vi "Delete Logged Files.vi"() -> ()   [LabVIEW 2019]
uses:
  <vilib>/Skyline/File/File/NI Skyline File.lvclass
  C:/Program Files (x86)/National Instruments/LabVIEW 2019/vi.lib/Skyline/File/Base/NI Skyline File Base.lvclass
  <vilib>/Skyline/File/Filter/Create Filter (Name).vi
  <vilib>/Skyline/File/Filter/Create Filter (Extension).vi
  <vilib>/Skyline/File/File/Query Files.vi
  <vilib>/Skyline/File/File/Delete (Multiple).vi
  <vilib>/Skyline/File/Filter/NI Skyline File Filter.lvclass
  <vilib>/Skyline/File/Base/NI Skyline File Base.lvclass
panel:
  out "Numeric":i32
  out "size(s)":i32
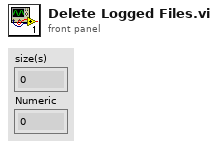
[diagram p1: front panel]
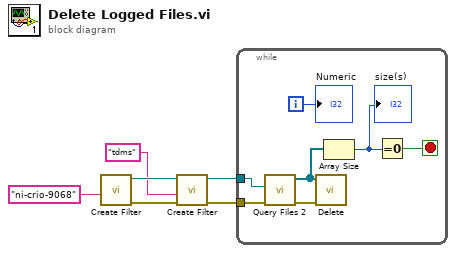
[diagram p0: block diagram]
diagram:
  n1 = call-poly <vilib>:"Create Filter.vi"("value"="ni-crio-9068") -> ("error out"=w5:errorcluster, "filter out"=w2:refnum<class "NI Skyline File Filter.lvclass">)  [unwired: 9 in]
  n2 = call-poly <vilib>:"Create Filter.vi"("error in (no error)"=w5, "value"="tdms", "filter in"=w2) -> ("error out"=w4:errorcluster, "filter out"=w3:refnum<class "NI Skyline File Filter.lvclass">)  [unwired: 7 in]
  n3 = while {
    tunnel: w4 -> [w12]
    tunnel: w3 -> [w11]
    i -> [w8]
    stop <- w9 stop-if-true
    n4 = call-poly <vilib>:"Query Files 2.vi"("error in (no error)"=w12, "filter"=w11) -> ("error out"=w13:errorcluster, "available files"=w7:refnum<class "NI Skyline File.lvclass">[])  [unwired: 7 in, 1 out]
    n5 = call-poly <vilib>:"Delete.vi"("error in (no error)"=w13, "files"=w7) -> ()  [unwired: 9 in, 1 out]
    n6 = Array Size(array=w7) -> (size(s)=w10:i32)
    "size(s)" <- w10
    n7 = Equal To 0?(x=w10) -> (x = 0?=w9:bool)
    "Numeric" <- w8
  }
